vi "FT conversion.vi"(2 "Control Box":T1={"Rotate & Translate"=FALSE, "rotation angle"=0.0, "Force Divider"=100.0, "Torque Divider"=1000.0}, 3 "CAN":u16[](array[numeric]), 4 "Bias":dbl[](array[numeric])=[0.0, 0.0, 0.0, 0.0, 0.0, 0.0]) -> (0 "ForceTorque":dbl[](array[numeric]), 1 "Unbiased DATA":dbl[](array[numeric]))   [LabVIEW 2011]
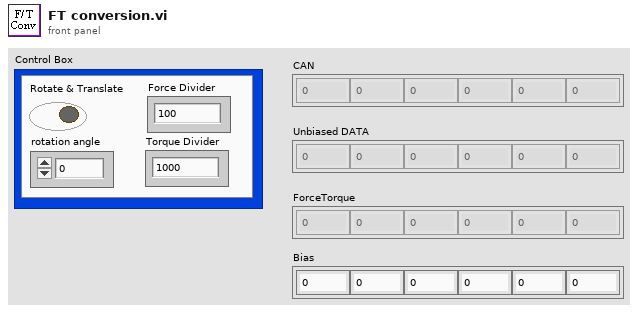
[diagram p1: front panel]
types:
  T1 = cluster{"Rotate & Translate":bool, "rotation angle":dbl, "Force Divider":dbl, "Torque Divider":dbl}
  T2 = cluster{"[0]":dbl, "[1]":dbl, "[2]":dbl, "[3]":dbl, "[4]":dbl, "[5]":dbl}
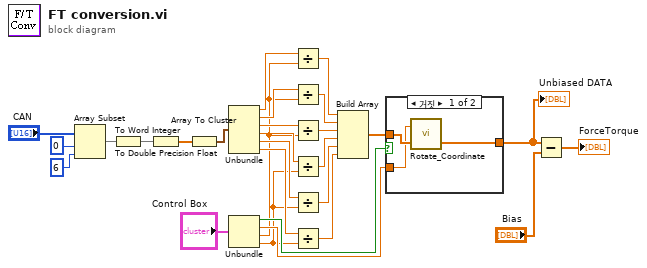
[diagram p0: block diagram]
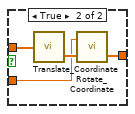
[diagram p2: hidden frame]
diagram:
  n1 = Array Subset(array="CAN", index=0 ("인덱스"), length=6 ("길이")) -> (w23:u16[])
  n2 = To Word Integer(number=w23) -> (16bit integer=w16:i16[])
  n3 = To Double Precision Float(number=w16) -> (double precision float=w15:dbl[])
  n4 = Array To Cluster(array=w15) -> (cluster=w14:T2)
  n5 = Unbundle(w14) -> ("[0]"=w13:dbl, "[1]"=w12:dbl, "[2]"=w11:dbl, "[3]"=w10:dbl, "[4]"=w9:dbl, "[5]"=w8:dbl)
  n6 = Unbundle("Control Box") -> ("Rotate & Translate"=w4:bool, "rotation angle"=w3:dbl, "Force Divider"=w2:dbl, "Torque Divider"=w1:dbl)
  n7 = Divide(x=w13, y=w2) -> (x/y=w17:dbl)
  n8 = Divide(x=w12, y=w2) -> (x/y=w18:dbl)
  n9 = Divide(x=w11, y=w2) -> (x/y=w19:dbl)
  n10 = Divide(x=w10, y=w1) -> (x/y=w20:dbl)
  n11 = Divide(x=w9, y=w1) -> (x/y=w21:dbl)
  n12 = Divide(x=w8, y=w1) -> (x/y=w22:dbl)
  n13 = Build Array(w17, w18, w19, w20, w21, w22) -> (w7:dbl[])
  n14 = case shown="거짓" w4 {
    tunnel: [w31 w35] -> w5
    tunnel: w7 -> [w30 w33]
    tunnel: w3 -> [w29 w32]
    frame False {
      n15 = call "Rotate_Coordinate.vi"("Input Data"=w30, "Rotation Angle"=w29) -> ("Rotated Data"=w31:dbl[])  [unwired: 1 out]
    }
    frame True {
      n16 = call "Translate_Coordinate.vi"("Input Data"=w33) -> ("Translated Data"=w34:dbl[])  [unwired: 1 out]
      n17 = call "Rotate_Coordinate.vi"("Input Data"=w34, "Rotation Angle"=w32) -> ("Rotated Data"=w35:dbl[])  [unwired: 1 out]
    }
  }
  "Unbiased DATA" <- w5
  n18 = Subtract(x=w5, y="Bias") -> (x-y=→"ForceTorque":dbl[])
